vi "DosageTimetable.vi"(0 "enable":bool, 1 "timetable":string[][](table) caption="Zeitplan", 5 "dosage":refnum<vi>, 7 "tank":refnum<vi>, 9 "volume":refnum<vi>, 11 "flowrate":refnum<vi>, 12 "error in":errorcluster) -> (15 "error out":errorcluster[](array[cluster]))   [LabVIEW 2011]
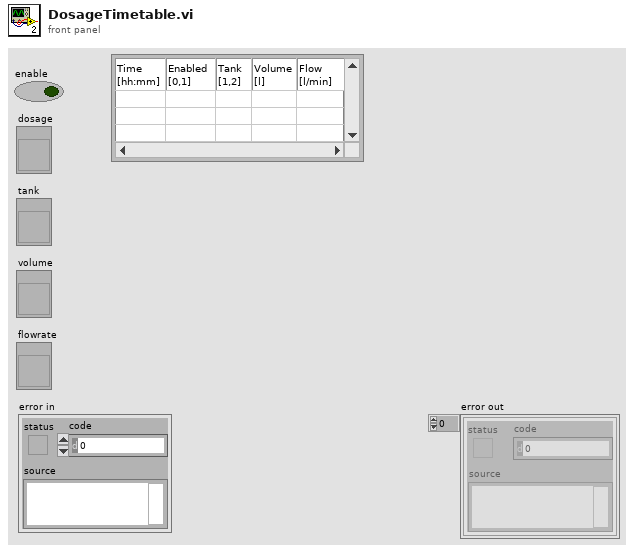
[diagram p1: front panel]
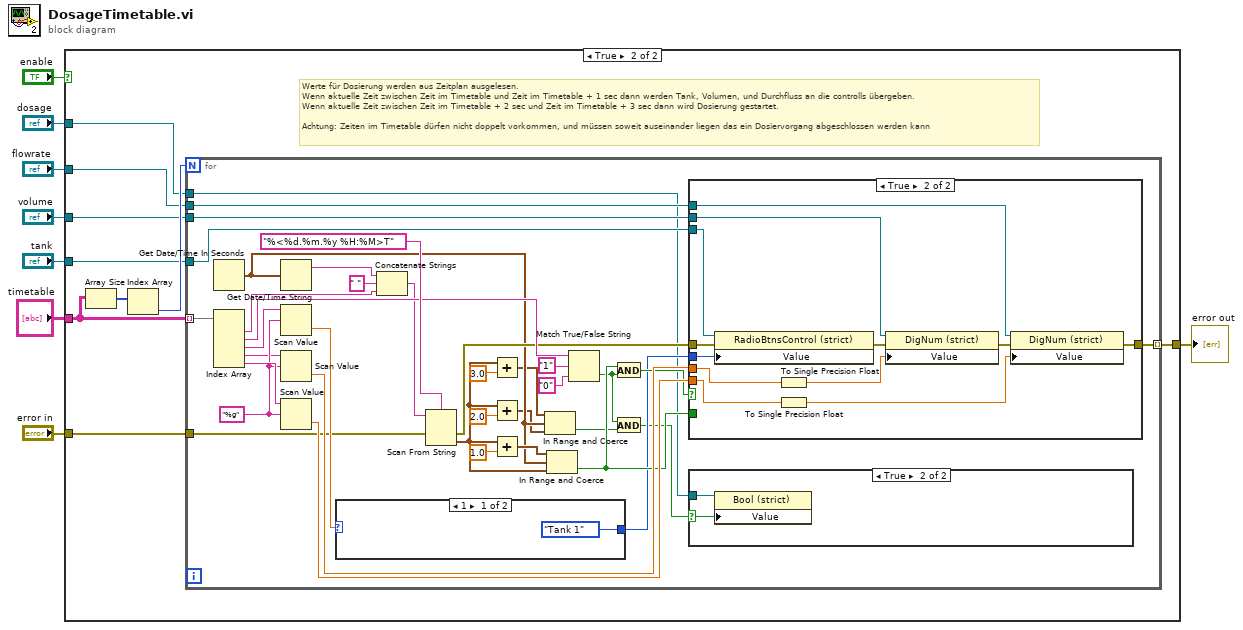
[diagram p0: block diagram]
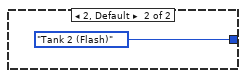
[diagram p4: hidden frame]
diagram:
  n1 = case shown="True" "enable" {
    tunnel: "timetable" -> [_ w17]
    tunnel: "dosage" -> [_ w14]
    tunnel: "tank" -> [_ w13]
    tunnel: "error in" -> [_ w12]
    tunnel: [_ w11] -> w6
    tunnel: "volume" -> [_ w10]
    tunnel: "flowrate" -> [_ w9]
    frame False {
    }
    frame True {
      # "Werte für Dosierung werden aus Zeitplan ausgelesen.\nWenn aktuelle Zeit zwischen Zeit im Timetable und Zeit im Timetable + 1 sec dann werden Tank, Volumen, und Durchfluss an die controlls übergeben.\nWenn aktuelle Zeit zwischen Zeit im Timetable + 2 sec und Zeit im Timetable + 3 sec dann wird Dosierung gestartet.\n\nAchtung: Zeiten im Timetable dürfen nicht doppelt vorkommen, und müssen soweit auseinander liegen das ein Dosiervorgang abgeschlossen werden kann"
      n2 = Array Size(array=w17) -> (size(s)=w16:i32[])
      n3 = Index Array(array=w16) -> (element=w15:i32)  [unwired: 1 in]
      n4 = for {
        N: w15 -> [_]
        tunnel: w17 -> [w54] mode=indexing
        tunnel: w14 -> [w20]
        tunnel: w13 -> [w33]
        tunnel: w12 -> [w32]
        tunnel: [w30] -> w11 mode=indexing
        tunnel: w10 -> [w29]
        tunnel: w9 -> [w28]
        w44 = "%g" ("format string")
        n5 = Get Date/Time In Seconds() -> (seconds since 1Jan1904=w27:timestamp)
        n6 = Index Array(array=w54) -> (element #1=w53:string, element #2=w49:string, element #3=w39:string, element #4=w38:string, element #5=w45:string)  [unwired: 5 in]
        n7 = Get Date/Time String(seconds (now)=w27) -> (date string=w37:string)  [unwired: 2 in, 1 out]
        n8 = Scan Value(string=w39, format string=w44) -> (value=w34:dbl)  [unwired: 1 in, 1 out]
        n9 = Scan Value(string=w38, format string=w44) -> (value=w46:dbl)  [unwired: 1 in, 1 out]
        n10 = Scan Value(string=w45, format string=w44) -> (value=w43:dbl)  [unwired: 1 in, 1 out]
        n11 = case shown="1" w34 {
          tunnel: [enum32{"Tank 1", "Tank 2 (Flash)"}."Tank 1" ("Zulauf") enum32{"Tank 1", "Tank 2 (Flash)"}."Tank 2 (Flash)" ("Zulauf")] -> w35
          frame 1 {
          }
          frame 2, Default {
          }
        }
        n12 = Concatenate Strings(w37, " " ("string"), w53) -> (w40:string)
        n13 = Scan From String(format string="%<%d.%m.%y %H:%M>T", input string=w40, error in=w32) -> (error out=w31:errorcluster, output 1=w25:timestamp)  [unwired: 2 in, 2 out]
        n14 = Add(x=w25, y=3.0) -> (x+y=w26:timestamp)
        n15 = Add(x=w25, y=2.0) -> (x+y=w19:timestamp)
        n16 = Add(x=w25, y=1.0) -> (x+y=w51:timestamp)
        n17 = In Range and Coerce(upper limit=w26, x=w27, lower limit=w19) -> (In Range?=w22:bool)  [unwired: 1 out]
        n18 = In Range and Coerce(upper limit=w51, x=w27, lower limit=w25) -> (In Range?=w41:bool)  [unwired: 1 out]
        n19 = Match True/False String(2:"0" ("false string"), 3:"1" ("true string"), 4:w49) -> (0:w21:bool)  [unwired: 1 out]
        n20 = And(x=w41, y=w21) -> (x .and. y?=w42:bool)
        n21 = And(x=w21, y=w22) -> (x .and. y?=w23:bool)
        n22 = case shown="True" w42 {
          tunnel: w41 -> [_ _]
          tunnel: w46 -> [_ w64]
          tunnel: w43 -> [_ w69]
          tunnel: w35 -> [_ w70]
          tunnel: w33 -> [_ w71]
          tunnel: w31 -> [w59 w63]
          tunnel: [w59 w60] -> w30
          tunnel: w29 -> [_ w66]
          tunnel: w28 -> [_ w65]
          frame False {
          }
          frame True {
            n23 = property on="Property Node" class="RadioBtnsControl (strict)"(reference=w71, error in=w63, "Value"=w70) -> (error out=w68:errorcluster)  [unwired: 1 out]
            n24 = To Single Precision Float(number=w64) -> (single precision float=w62:sgl)
            n25 = To Single Precision Float(number=w69) -> (single precision float=w61:sgl)
            n26 = property on="Property Node" class="DigNum (strict)"(reference=w66, error in=w68, "Value"=w62) -> (error out=w67:errorcluster)  [unwired: 1 out]
            n27 = property on="Property Node" class="DigNum (strict)"(reference=w65, error in=w67, "Value"=w61) -> (error out=w60:errorcluster)  [unwired: 1 out]
          }
        }
        n28 = case shown="True" w23 {
          selector: w23 -> [_ w55]
          tunnel: w20 -> [_ w56]
          frame False {
          }
          frame True {
            n29 = property on="Property Node" class="Bool (strict)"(reference=w56, "Value"=w55) -> ()  [unwired: 1 in, 2 out]
          }
        }
      }
    }
  }
  "error out" <- w6
